vi "Update Tree Item Symbol and Clolor.vi"(7 "Tree Refnum":refnum<vi>, 8 "error in":errorcluster, 11 "Tree Control Items":T1(array[cluster])) -> (0 "error out":errorcluster, 3 "Tree Control ItemsOut":T1(array[cluster]))   [LabVIEW 2019]
doc: "All Rights Reserved © 2017 SyncSols"
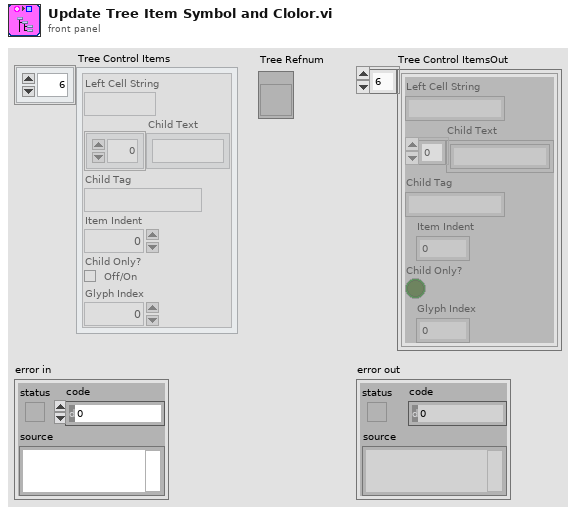
[diagram p1: front panel]
types:
  T1 = cluster{"Left Cell String":string, "Child Text":string[], "Child Tag":string, "Item Indent":i32, "Child Only?":bool, "Glyph Index":i32}[]
  T2 = cluster{"Left Cell String":string, "Child Text":string[], "Child Tag":string, "Item Indent":i32, "Child Only?":bool, "Glyph Index":i32}
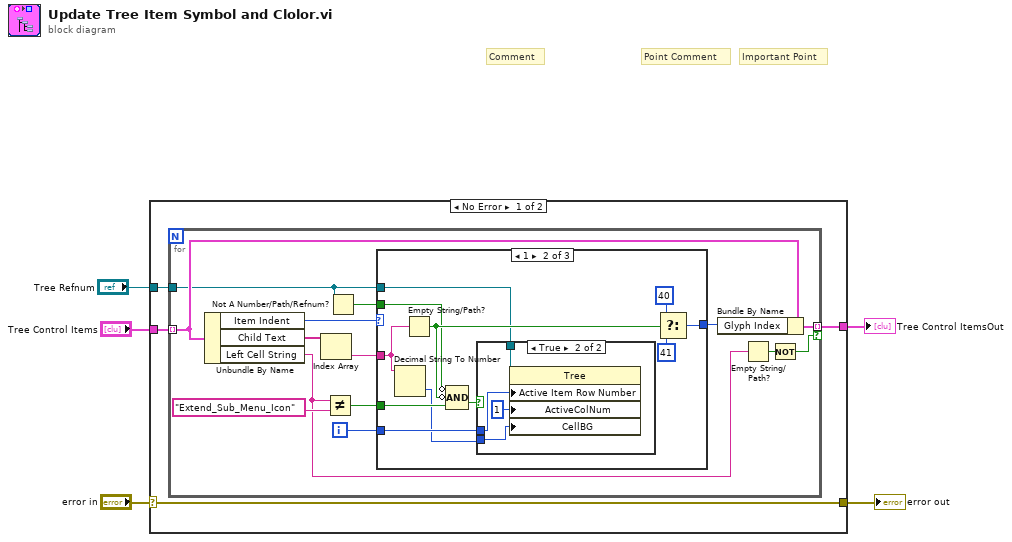
[diagram p0: block diagram]
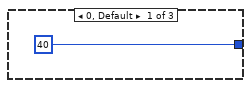
[diagram p2: hidden frame]
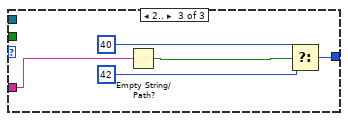
[diagram p4: hidden frame]
diagram:
  # "Important Point"
  # "Point Comment"
  # "Comment"
  n1 = case shown="No Error" "error in" {
    selector: "error in" -> [w9 w46]
    tunnel: [w9 w46] -> w5
    tunnel: "Tree Control Items" -> [w8 w45]
    tunnel: [w7 w45] -> w2
    tunnel: "Tree Refnum" -> [w6 _]
    frame No Error {
      n2 = for {
        tunnel: w8 -> [w22] mode=indexing
        tunnel: [w20] -> w7 mode=indexing if=w10
        tunnel: w6 -> [w14]
        i -> [w15]
        n3 = Unbundle By Name(w22) -> ("Item Indent"=w23:i32, "Child Text"=w19:string[], "Left Cell String"=w12:string)
        n4 = Index Array(array=w19) -> (element=w18:string)  [unwired: 1 in]
        n5 = Not Equal?(x=w12, y="Extend_Sub_Menu_Icon") -> (x != y?=w16:bool)
        n6 = Not A Number/Path/Refnum?(number/path/refnum=w14) -> (NaN/Path/Refnum?=w13:bool)
        n7 = case shown="1" w23 {
          tunnel: [40 ("Glyph Index") w35 w44] -> w21
          tunnel: w18 -> [_ w32 w41]
          tunnel: w16 -> [_ w31 _]
          tunnel: w14 -> [_ w28 _]
          tunnel: w15 -> [_ w27 _]
          tunnel: w13 -> [_ w25 _]
          frame 0, Default {
          }
          frame 1 {
            n8 = Decimal String To Number(string=w32) -> (number=w26:i32)  [unwired: 2 in, 1 out]
            n9 = Empty String/Path?(string/path=w32) -> (empty?=w29:bool)
            n10 = Compound Arithmetic op=AND(invert w25, invert w29, w31) -> (w30:bool)
            n11 = case shown="True" w30 {
              tunnel: w28 -> [_ w39]
              tunnel: w27 -> [_ w38]
              tunnel: w26 -> [_ w36]
              frame False {
              }
              frame True {
                n12 = property class="Tree"(reference=w39, "Active Item Row Number"=w38, "ActiveColNum"=1 ("Active Cell:Active Column Number"), "CellBG"=w36) -> ()  [unwired: 1 in, 2 out]
              }
            }
            n13 = Select(t=40 ("Glyph Index"), s=w29, f=41 ("Glyph Index")) -> (s? t:f=w35:i32)
          }
          frame 2.. {
            n14 = Empty String/Path?(string/path=w41) -> (empty?=w40:bool)
            n15 = Select(t=40 ("Glyph Index"), s=w40, f=42 ("Glyph Index")) -> (s? t:f=w44:i32)
          }
        }
        n16 = Bundle By Name(cluster=w22, "Glyph Index"=w21) -> (w20:T2)
        n17 = Empty String/Path?(string/path=w12) -> (empty?=w11:bool)
        n18 = Not(x=w11) -> (.not. x?=w10:bool)
      }
    }
    frame Error {
    }
  }
  "error out" <- w5
  "Tree Control ItemsOut" <- w2
